vi "dfd_Lattice Allpass Normalization (Basic).vi"(7 "scale type":T1, 10 "coefficients k":dbl[](array[numeric]) format="%.2f", 11 "x":dbl[](array[numeric])) -> (2 "norm":dbl[](array[numeric]) format="%.2f", 3 "y":dbl[](array[numeric]))   [LabVIEW 2017, in "NI_DigFilter_FXP.lvlib"]
uses:
  <vilib>/addons/Digital Filter Design/NI_DigFilter_FXP.lvlib
  <vilib>/addons/Digital Filter Design/_Objects.llb/DFD Coef Norm Type.ctl
  <vilib>/addons/Digital Filter Design/NI_DigFilterLicensed.lvlib
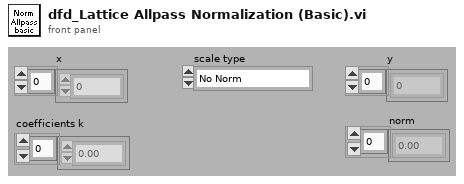
[diagram p1: front panel]
types:
  T1 = typedef "NI_DigFilterLicensed.lvlib/DFD Coef Norm Type.ctl" = enum16{"No Norm", "Time Domain 1-Norm", "Time Domain 2-Norm", "Time Domain Inf-Norm"}
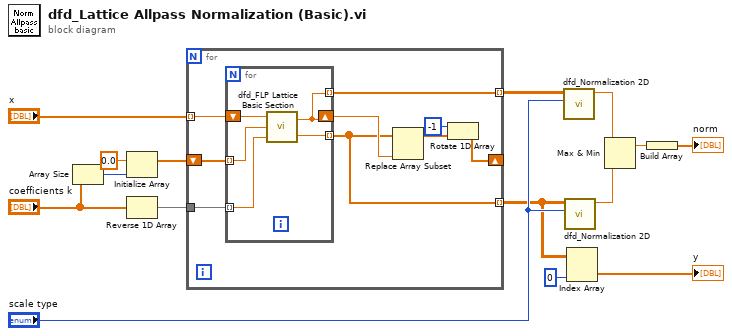
[diagram p0: block diagram]
diagram:
  n1 = Array Size(array="coefficients k") -> (size(s)=w13:i32)
  n2 = Initialize Array(0.0 ("element"), w13) -> (w15:dbl[])
  n3 = Reverse 1D Array(array="coefficients k") -> (reversed array=w12:dbl[])
  n4 = for {
    tunnel: w12 -> [w24]
    shift-right: [w19] -> _
    shift-left: w15 -> [w23]
    tunnel: [w16] -> w4 mode=indexing
    tunnel: [w22] -> w5 mode=indexing
    tunnel: "x" -> [w21] mode=indexing
    n5 = for {
      shift-right: [w27] -> w17
      shift-left: w21 -> [w29]
      tunnel: w24 -> [w28] mode=indexing
      tunnel: [w27] -> w22 mode=indexing
      tunnel: w23 -> [w26] mode=indexing
      tunnel: [w25] -> w16 mode=indexing
      n6 = call <vilib>:"dfd_FLP Lattice Basic Section.vi"("k(m)"=w28, "w(m-1)"=w26, "x(m)"=w29) -> ("w(m)"=w25:dbl, "x(m-1)"=w27:dbl)
    }
    n7 = Replace Array Subset(array=w16, new element=w17) -> (w18:dbl[])  [unwired: 1 in]
    n8 = Rotate 1D Array(1:w18, 2:-1 ("n")) -> (0:w19:dbl[])
  }
  n9 = call <vilib>:"dfd_Normalization 2D.vi"("scale type"="scale type", "2D Array (col-major)"=w5) -> ("max norm"=w2:dbl)  [unwired: 1 in, 8 out]
  n10 = call <vilib>:"dfd_Normalization 2D.vi"("scale type"="scale type", "2D Array (col-major)"=w4) -> ("max norm"=w1:dbl)  [unwired: 1 in, 8 out]
  n11 = Index Array(array=w4, index (col)=0 ("index (row)")) -> (element=→"y":dbl[])  [unwired: 1 in]
  n12 = Max & Min(x=w2, y=w1) -> (max(x,y)=w8:dbl)  [unwired: 1 out]
  n13 = Build Array(w8) -> (→"norm":dbl[])
